vi "数字量输入统计结果.vi"() -> ()   [LabVIEW 2010]
uses:
  全局量/全局_配置.vi
  全局量/自动测试结果.vi
panel:
  in  "余数":i32
  out "数据组数":i32
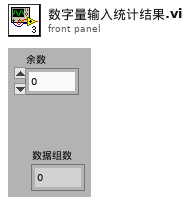
[diagram p1: front panel]
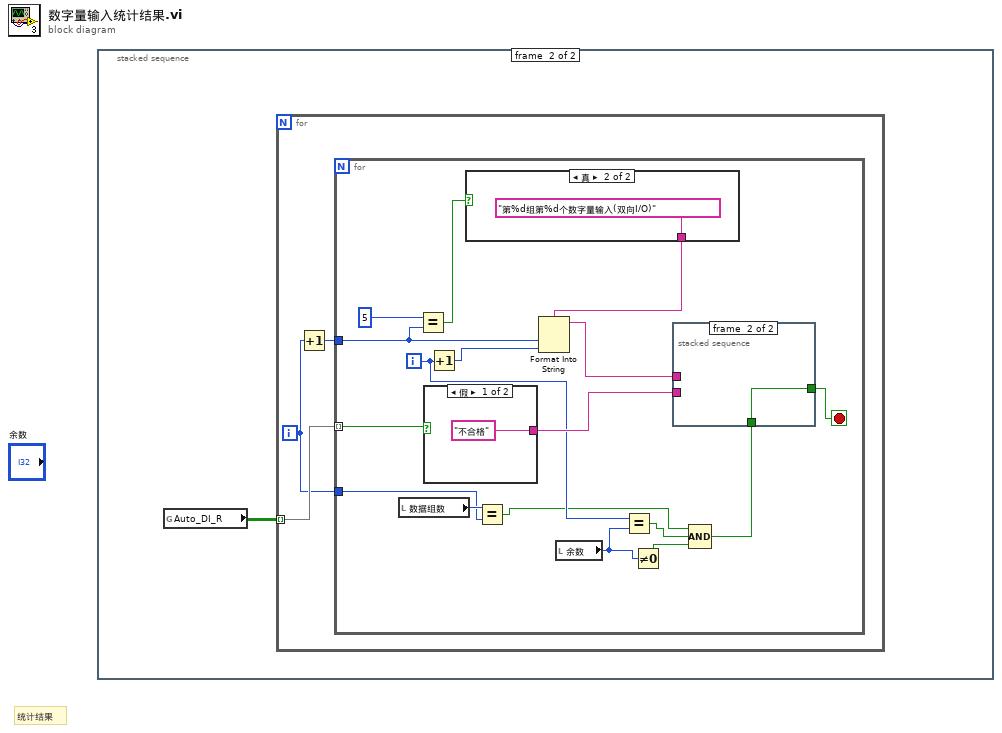
[diagram p0: block diagram]
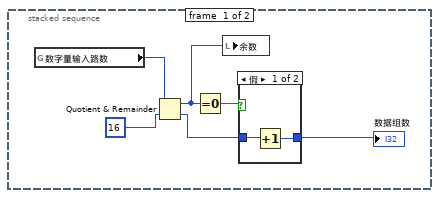
[diagram p2: hidden frame]
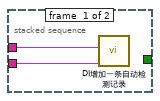
[diagram p4: hidden frame]
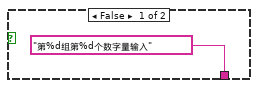
[diagram p5: hidden frame]
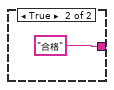
[diagram p6: hidden frame]
diagram:
  # "统计结果"
  n1 = stacked-sequence {
    frame #0 {
      n2 = global read "全局_配置.vi" "数字量输入路数"() -> (w3:i32)
      n3 = Quotient & Remainder(x=w3, y=16) -> (x-y*floor(x/y)=w1:i32, floor(x/y)=w5:i32)
      n4 = Equal To 0?(x=w1) -> (x = 0?=w6:bool)
      n5 = local write "余数"(w1) -> ()
      n6 = case shown="假" w6 {
        tunnel: w5 -> [w8 w9]
        tunnel: [w7 w9] -> w2
        frame False {
          n7 = Increment(x=w8) -> (x+1=w7:i32)
        }
        frame True {
        }
      }
      "数据组数" <- w2
    }
    frame #1 {
      n8 = global read "自动测试结果.vi" "Auto_DI_R"() -> (w10:bool[][])
      n9 = for {
        tunnel: w10 -> [w13] mode=indexing
        i -> [w11]
        n10 = Increment(x=w11) -> (x+1=w12:i32)
        n11 = for {
          tunnel: w13 -> [w28] mode=indexing
          tunnel: w12 -> [w26]
          tunnel: w11 -> [w21]
          i -> [w20]
          stop <- w15 stop-if-true
          n12 = local read "数据组数"() -> (w22:i32)
          n13 = Equal?(x=5, y=w26) -> (x = y?=w24:bool)
          n14 = case shown="假" w28 {
            tunnel: ["不合格" "合格"] -> w27
            frame False {
            }
            frame True {
            }
          }
          n15 = Increment(x=w20) -> (x+1=w30:i32)
          n16 = case shown="真" w24 {
            tunnel: ["第%d组第%d个数字量输入" "第%d组第%d个数字量输入(双向I/O)"] -> w23
            frame False {
            }
            frame True {
            }
          }
          n17 = Equal?(x=w22, y=w21) -> (x = y?=w18:bool)
          n18 = Format Into String(format string=w23, w26, w30) -> (resulting string=w29:string)  [unwired: 2 in, 1 out]
          n19 = local read "余数"() -> (w19:i32)
          n20 = Equal?(x=w20, y=w19) -> (x = y?=w17:bool)
          n21 = Not Equal To 0?(x=w19) -> (x != 0?=w16:bool)
          n22 = Compound Arithmetic op=AND(w18, w17, w16) -> (w14:bool)
          n23 = stacked-sequence {
            tunnel: w29 -> [w32 _]
            tunnel: w27 -> [w31 _]
            tunnel: [_ w33] -> w15
            tunnel: w14 -> [_ w33]
            frame #0 {
              n24 = call "DI增加一条自动检测记录.vi"("测试结果"=w31, "测试内容"=w32) -> ()  [unwired: 10 in]
            }
            frame #1 {
            }
          }
        }
      }
    }
  }
